vi "Measure Simu.vi"(0 "OnOff.ACT":bool, 1 "ErrorAcknowledge.ACT":bool, 2 "Iteration Interval (s)":dbl, 3 "Channels In":T2(array[cluster]), 6 "Current Feedback In":dbl[](array[numeric]), 7 "Voltage Feedback In":dbl[](array[numeric]), 10 "Power Feedback In":dbl[](array[numeric]), 11 "Error Feedback In":bool[](array[boolean])) -> (8 "Current Feedback Out":dbl[](array[numeric]), 9 "Voltage Feedback Out":dbl[](array[numeric]), 12 "Power Feedback out":dbl[](array[numeric]), 13 "Error Feedback Out":bool[](array[boolean]), 14 "Channels Out":T1(array[cluster]), 15 "Error Out":bool[](array[boolean]))   [LabVIEW 2023]
uses:
  Capabilities/Capabilities/High Level Capabilities/Cycler Cluster/Producer Ch.ctl
  Capabilities/Capabilities/High Level Capabilities/Cycler Cluster/Cycler Cluster.lvclass
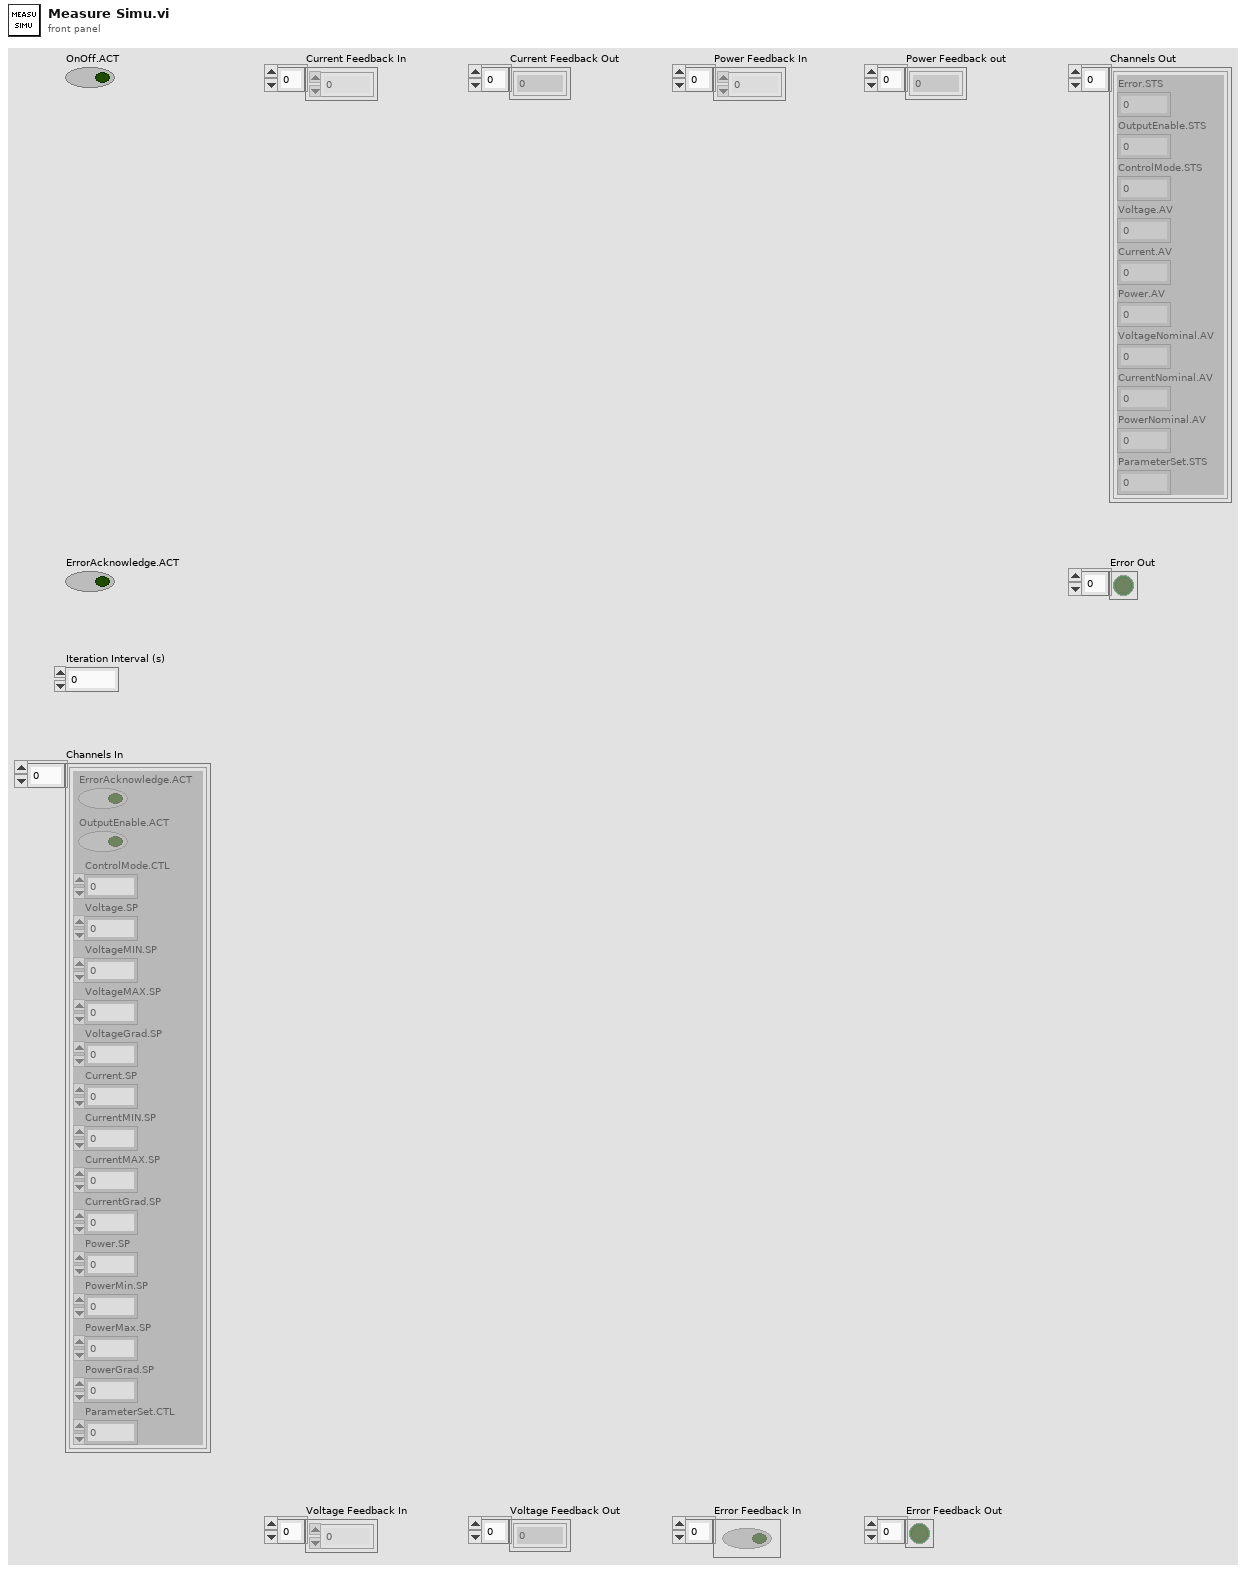
[diagram p1: front panel]
types:
  T1 = cluster{"Error.STS":i32, "OutputEnable.STS":i32, "ControlMode.STS":u16, "Voltage.AV":dbl, "Current.AV":dbl, "Power.AV":dbl, "VoltageNominal.AV":dbl, "CurrentNominal.AV":dbl, "PowerNominal.AV":dbl, "ParameterSet.STS":i32}[]
  T2 = cluster{"ErrorAcknowledge.ACT":bool, "OutputEnable.ACT":bool, "ControlMode.CTL":u16, "Voltage.SP":dbl, "VoltageMIN.SP":dbl, "VoltageMAX.SP":dbl, "VoltageGrad.SP":dbl, "Current.SP":dbl, "CurrentMIN.SP":dbl, "CurrentMAX.SP":dbl, "CurrentGrad.SP":dbl, "Power.SP":dbl, "PowerMin.SP":dbl, "PowerMax.SP":dbl, "PowerGrad.SP":dbl, "ParameterSet.CTL":i32}[]
  T3 = typedef "Cycler Cluster.lvclass/Producer Ch.ctl" = cluster{"Error.STS":i32, "OutputEnable.STS":i32, "ControlMode.STS":u16, "Voltage.AV":dbl, "Current.AV":dbl, "Power.AV":dbl, "VoltageNominal.AV":dbl, "CurrentNominal.AV":dbl, "PowerNominal.AV":dbl, "ParameterSet.STS":i32}
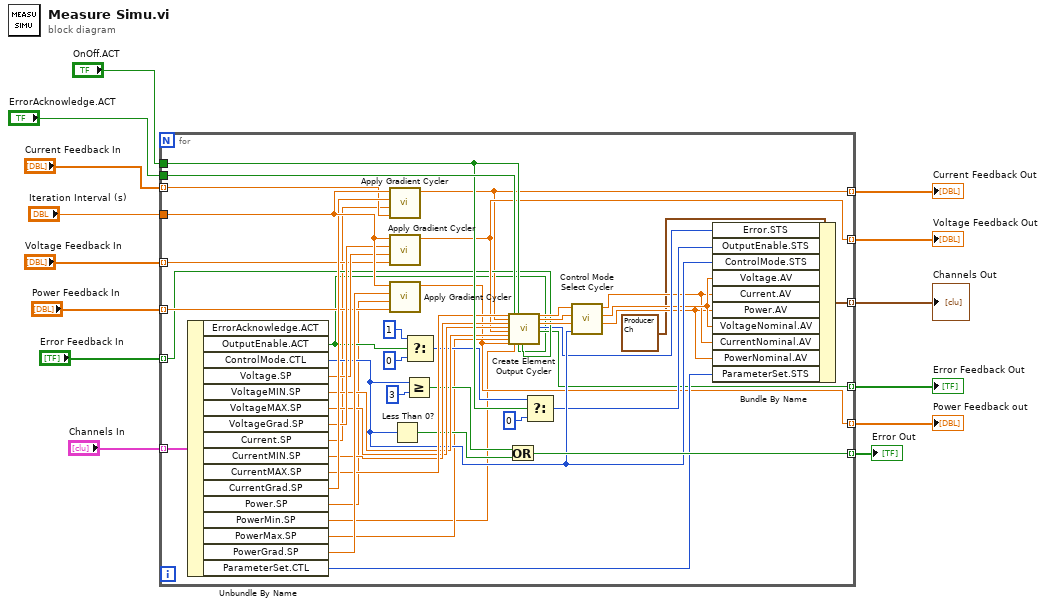
[diagram p0: block diagram]
diagram:
  n1 = for {
    tunnel: "ErrorAcknowledge.ACT" -> [w56]
    tunnel: "OnOff.ACT" -> [w55]
    tunnel: "Iteration Interval (s)" -> [w54]
    tunnel: "Channels In" -> [w29] mode=indexing
    tunnel: [w42] -> w2 mode=indexing
    tunnel: [w36] -> w5 mode=indexing
    tunnel: "Voltage Feedback In" -> [w35] mode=indexing
    tunnel: "Current Feedback In" -> [w34] mode=indexing
    tunnel: [w30] -> w6 mode=indexing
    tunnel: "Power Feedback In" -> [w33] mode=indexing
    tunnel: [w16] -> w4 mode=indexing
    tunnel: [w20] -> w3 mode=indexing
    tunnel: "Error Feedback In" -> [w32] mode=indexing
    tunnel: [w22] -> w1 mode=indexing
    n2 = Unbundle By Name(w29) -> ("OutputEnable.ACT"=w19:bool, "ControlMode.CTL"=w37:u16, "Voltage.SP"=w46:dbl, "VoltageMIN.SP"=w47:dbl, "VoltageMAX.SP"=w48:dbl, "VoltageGrad.SP"=w49:dbl, "Current.SP"=w31:dbl, "CurrentMIN.SP"=w50:dbl, "CurrentMAX.SP"=w51:dbl, "CurrentGrad.SP"=w52:dbl, "Power.SP"=w18:dbl, "PowerMin.SP"=w15:dbl, "PowerMax.SP"=w17:dbl, "PowerGrad.SP"=w53:dbl, "ParameterSet.CTL"=w23:i32)  [unwired: 1 out]
    n3 = call "Apply Gradient Cycler.vi"("Reminder"=w34, "Setpoint"=w31, "Gradient"=w52, "Iteration Interval"=w54) -> ("Current Setpoint"=w30:dbl)  [unwired: 7 in]
    n4 = call "Apply Gradient Cycler.vi"("Reminder"=w35, "Setpoint"=w46, "Gradient"=w49, "Iteration Interval"=w54) -> ("Current Setpoint"=w36:dbl)  [unwired: 7 in]
    n5 = call "Apply Gradient Cycler.vi"("Reminder"=w33, "Setpoint"=w18, "Gradient"=w53, "Iteration Interval"=w54) -> ("Current Setpoint"=w16:dbl)  [unwired: 7 in]
    n6 = Less Than 0?(x=w37) -> (x < 0?=w44:bool)
    n7 = Greater Or Equal?(x=w37, y=u16 3) -> (x >= y?=w45:bool)
    n8 = Select(t=1, s=w19, f=0) -> (s? t:f=w38:i32)
    n9 = Or(x=w45, y=w44) -> (x .or. y?=w42:bool)
    n10 = call "Create Element Output Cycler.vi"("Current Max SP"=w51, "Current In"=w30, "Current Min SP"=w50, "Voltage Max SP"=w48, "Voltage In"=w36, "Voltage Min SP"=w47, "Power Max SP"=w17, "Power In"=w16, "Error ACT"=w56, "Power Min SP"=w15, "OnOff ACT"=w55, "Output Enable ACT"=w19, "Feedback In"=w32) -> ("Current Out"=w59:dbl, "Voltage Out"=w58:dbl, "Power Out"=w57:dbl, "Error Channels"=w28:i32, "Feedback Out"=w20:bool)  [unwired: 10 in]
    n11 = Select(t=w38, s=w55, f=0) -> (s? t:f=w27:i32)
    n12 = call "Control Mode Select Cycler.vi"("Control Mode Read"=w37, "Power Read"=w57, "Voltage Read"=w58, "Current Read"=w59) -> ("Power Write"=w24:dbl, "Voltage Write"=w26:dbl, "Current Write"=w25:dbl)  [unwired: 5 in]
    n13 = Bundle By Name(cluster=T3 {"Error.STS"=0, "OutputEnable.STS"=0, "ControlMode.STS"=0, "Voltage.AV"=0.0, "Current.AV"=0.0, "Power.AV"=0.0, "VoltageNominal.AV"=0.0, "CurrentNominal.AV"=0.0, "PowerNominal.AV"=0.0, "ParameterSet.STS"=0} ("Producer Ch"), "Error.STS"=w28, "OutputEnable.STS"=w27, "ControlMode.STS"=w37, "Voltage.AV"=w26, "Current.AV"=w25, "Power.AV"=w24, "VoltageNominal.AV"=w26, "CurrentNominal.AV"=w25, "PowerNominal.AV"=w24, "ParameterSet.STS"=w23) -> (w22:T3)
  }
  "Current Feedback Out" <- w6
  "Voltage Feedback Out" <- w5
  "Power Feedback out" <- w4
  "Error Feedback Out" <- w3
  "Error Out" <- w2
  "Channels Out" <- w1
